vi "VI FID Konfig.vi"() -> ()   [LabVIEW 2020, in "ABB-EL3000.lvlib" / "FID.lvlib"]
uses:
  FID.lvlib
  CalGas Aufschaltung/Aufschaltung CalGas_ANZEIGE.ctl
  Visualisierungs Elemente/Auswahlfeld.ctl
  FID Kalibrierung/FID Kal Komponente.ctl
  Modus.ctl
  Visualisierungs Elemente/Zahlen-Ausgabefeld.ctl
  FID Kalibrierung/Aktionen FID Kal Komponente.ctl
  CalGas Aufschaltung/FGV CalGas Aktionen.ctl
  FT-IR/FGV FT-IR Gasliste Aktionen.ctl
  Aktion FGV Messwerte_F.ctl
  Messdaten/Aktionen FGV Messdaten.ctl
  Allgemeine VI/FGV Uras26 Aktion.ctl
  FID Kalibrierung/Aktion FID Allgemeindaten.ctl
  Aktion STY_MES.ctl
  Passwortverwaltung/FGV Passwort Aktion.ctl
  Analysator Definition/FGV Analysator Definition Aktionen.ctl
  FID Kalibrierung/FID Kalibrieren.ctl
  FT-IR/FGV FT-IR Parameter.vi
  Hangup Check/Hangup Main.vi
  Messdaten/Messdaten.lvlib
  CalGas Aufschaltung/CalGas Aufschaltung.lvlib
  FT-IR/FT-IR.lvlib
  Allgemein/allgemeine Sub-VIs.lvlib
  Analysator Definition/Analysator Definition.lvlib
  Passwortverwaltung/Passwort.lvlib
  FID Kalibrierung/FID Kalibrierung.lvlib
  Allgemeine VI/Allgemeine VI.lvlib
  Grafik/Grafik.lvlib
  Hangup Check/Hangup Check.lvlib
panel:
  out "Wert CH4 2":sgl caption="Kal. Wert THC:" format="%.1f"
  in  "Hang-Up Check":bool caption="Endpunkt"
  out "Roh Wert THC:":T1 format="%.1f"
  out "Response":string
  in  "Switching time":sgl caption="sec" min=0 format="%#.0f"
  in  "Mode":T2
  out "THC":string
  out "Mwert CH4":sgl format="%.1f"
  out "PMwert CH4":sgl format="%.1f"
  out "Wert CH4":sgl caption="Konzentration" format="%.1f"
  out "Graph CH4":waveform(dbl)[](graph)
  out "CH4":string
  out "Mwert 1THC":sgl format="%.1f"
  out "PMwert 1THC":sgl format="%.1f"
  out "Wert1 THC":sgl caption="Konzentration" format="%.1f"
  out "Graph1THC":waveform(dbl)[](graph)
  out "NMHC":string
  out "Mwert NMHC":sgl format="%.1f"
  out "PMwert NMHC":sgl format="%.1f"
  out "Wert NMHC":sgl caption="Konzentration" format="%.1f"
  out "MNHC":waveform(dbl)[](graph)
  in  "Endpunkt THC":bool
  in  "0-Punkt THC":bool
  in  "Kalidaten":bool
  in  "Endpunkt":bool
  in  "0-Punkt":bool
  in  "HC Messbereich":u16(ring)
  out "Wartungsbedarf":bool
  out "Funktionskontrolle":bool
  out "Ausfall":bool
  out "Flow Stellg":sgl caption="%" format="%#.1g"
  out "Durchfluss:":sgl format="%#.1f"
  out "Druck MGA":sgl caption="%" format="%#.1f"
  out "Druck MGE:":sgl caption="%" format="%#.1f"
  out "Brenngas:":sgl caption="%" format="%#.1f"
  out "Brennluft:":sgl caption="%" format="%#.1f"
  out "Messgaseingang":sgl caption="%" format="%#.1f"
  out "Detektor":sgl caption="%" format="%#.1f"
  out "Druck Messgasausgang:":sgl format="%#.1f"
  out "Druck Messgaseingang:":sgl format="%#.1f"
  out "Druck Brenngas H2/He:":sgl format="%#.1f"
  out "Druck Brennluft:":sgl format="%#.1f"
  out "Temperatur Flamme:":sgl format="%#.1f"
  out "Temperatur Messgaseingang:":sgl format="%#.1f"
  out "Temperatur Detektor:":sgl format="%.1f"
  in  "FID kalibrieren mit:":T3
  in  "Aufschaltung CalGas":T4 {"Aufschaltpunkt" items=["Filterblock", "Analysator direkt", "PNS", "Entnahme", "Gasdivider"]; "Kalibriergas" items=["Stickstoff"]}
  # "Konfiguration FID"
  # "Grafik"
  # "Hilfsgrößen"
  # "Temperaturen"
  # "Stellgröße"
  # "°C"
  # "°C"
  # "°C"
  # "hPa"
  # "hPa"
  # "hPa"
  # "hPa"
  # "l/h"
  # "Aufschaltung Kalibriergas"
  # "Kalibriergas"
  # "Aufschaltpunkt"
  # "Analysator"
  # "Modus (cutter)"
  # "±"
  # "x"
  # "±"
  # "x"
  # "±"
  # "x"
  # "Durchfluss"
  # "Druck"
  # "STATUS"
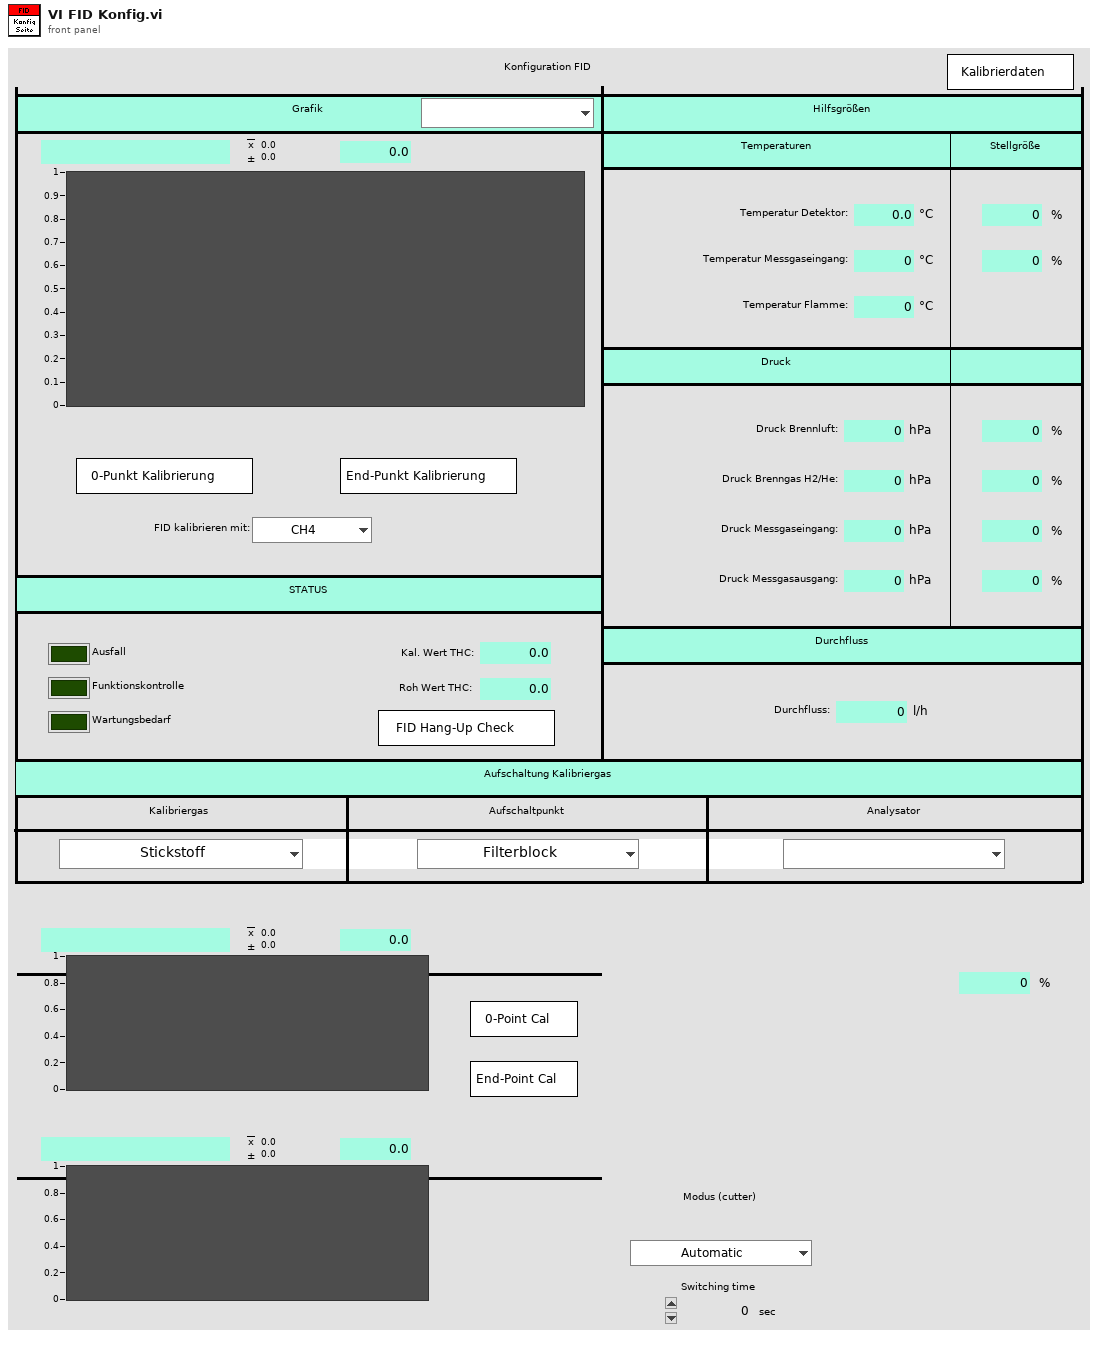
[diagram p1: front panel]
types:
  T1 = typedef "Zahlen-Ausgabefeld.ctl" = sgl
  T2 = typedef "ABB-EL3000.lvlib/FID.lvlib/Modus.ctl" = enum16{"Automatic", "CH4", "THC", "Efficienty measure", "Switching time"}
  T3 = typedef "ABB-EL3000.lvlib/FID.lvlib/FID Kalibrierung.lvlib/FID Kal Komponente.ctl" = enum16{"CH4", "C3H8"}
  T4 = typedef "CalGas Aufschaltung.lvlib/Aufschaltung CalGas_ANZEIGE.ctl" = cluster{"Kalibriergas":T5, "Aufschaltpunkt":T5, "Analysator":T5}
  T5 = typedef "Auswahlfeld.ctl" = u16
  T6 = typedef "ABB-EL3000.lvlib/FID.lvlib/FID Kalibrierung.lvlib/Aktionen FID Kal Komponente.ctl" = enum16{"lesen", "setzen", "laden", "speichern", "LIN"}
  T7 = typedef "ABB-EL3000.lvlib/FID.lvlib/FID Kalibrierung.lvlib/Aktion FID Allgemeindaten.ctl" = enum16{"lesen", "Mod", "Time", "laden", "speichern"}
  T8 = typedef "FT-IR.lvlib/FGV FT-IR Gasliste Aktionen.ctl" = enum16{"lesen", "Gasliste FT-IR", "Gasliste ausgelesen", "laden", "speichern", "löschen"}
  T9 = typedef "CalGas Aufschaltung.lvlib/FGV CalGas Aktionen.ctl" = enum16{"lesen", "Analysator Auswahl", "Def.CalGas", "Aufschaltung CalGas", "laden", "speichern", "KAL extrahieren"}
  T10 = typedef "String - Ausgabefeld.ctl" = string
  T11 = typedef "CalGas Aufschaltung.lvlib/Aufschaltung CalGas.ctl" = cluster{"Kalibriergas":T5, "Aufschaltpunkt":T12, "Analysator":T13}
  T12 = typedef "CalGas Aufschaltung.lvlib/Auswahl Aufschaltpunkt.ctl" = enum16{"über Filterblock", "Analysator direkt", "über PNS", "Entnahme", "Gasdivider"}
  T13 = typedef "CalGas Aufschaltung.lvlib/Auswahl Analysator.ctl" = enum16{"FT-IR", "FID", "PMA", "PMA/FID/FT-IR"}
  T14 = typedef "CalGas Aufschaltung.lvlib/Definition CalGas Anzeige.ctl" = cluster{"Namen":T15, "Werte":T17, "Werte 2":T17, "Einheit":T19, "Messbereiche":T20}
  T15 = typedef "CalGas Aufschaltung.lvlib/CalGas-Namen.ctl" = cluster{"Name":T16, "Name 2":T16, "Name 3":T16, "Name 4":T16, "Name 5":T16, "Name 6":T16, "Name 7":T16, "Name 8":T16, "Name 9":T16, "Name 10":T16, "Name 11":T16, "Name 12":T16}
  T16 = typedef "String - Eingabefeld.ctl" = string
  T17 = typedef "CalGas Aufschaltung.lvlib/CalGas-Werte.ctl" = cluster{"Konzentration 1":T18, "Konzentration 2":T18, "Konzentration 3":T18, "Konzentration 4":T18, "Konzentration 5":T18, "Konzentration 6":T18, "Konzentration 7":T18, "Konzentration 8":T18, "Konzentration 9":T18, "Konzentration 10":T18, "Konzentration 11":T18, "Konzentration 12":T18}
  T18 = typedef "Zahlen-Eingabefeld.ctl" = sgl
  T19 = typedef "CalGas Aufschaltung.lvlib/CalGas-Einheit.ctl" = cluster{"Einheit 1":T5, "Einheit 2":T5, "Einheit 3":T5, "Einheit 4":T5, "Einheit 5":T5, "Einheit 6":T5, "Einheit 7":T5, "Einheit 8":T5, "Einheit 9":T5, "Einheit 10":T5, "Einheit 11":T5, "Einheit 12":T5}
  T20 = typedef "CalGas Aufschaltung.lvlib/CalGas-Messbereiche.ctl" = cluster{"Messbereich 1":T5, "Messbereich 2":T5, "Messbereich 3":T5, "Messbereich 4":T5, "Messbereich 5":T5, "Messbereich 6":T5, "Messbereich 7":T5, "Messbereich 8":T5, "Messbereich 9":T5, "Messbereich 10":T5, "Messbereich 11":T5, "Messbereich 12":T5}
  T21 = typedef "Messdaten.lvlib/Aktionen FGV Messdaten.ctl" = enum16{"lesen", "schreiben", "löschen", "Mittelwerte", "Komponente"}
  T22 = typedef "ABB-EL3000.lvlib/Allgemeine VI.lvlib/FGV Uras26 Aktion.ctl" = enum16{"lesen", "CAL-Daten laden", "Messen", "Kalibrieren vorbereiten", "Kalibrieren", "CAL-Daten speichern", "Toleranz schreiben", "CAL-Daten kopieren"}
  T23 = typedef "ABB-EL3000.lvlib/FID.lvlib/Aktion FGV Messwerte_F.ctl" = enum16{"lesen", "Messwerte", "Messbereich", "Status", "Diagnose Werte"}
  T24 = typedef "Aktion STY_MES.ctl" = enum16{"lesen", "setze STY", "setze MES", "MODBUS schreiben"}
  T25 = typedef "Passwort.lvlib/FGV Passwort Aktion.ctl" = enum16{"prüfen", "setzen", "Initialisieren", "PW speichern", "lesen", "PW Änderung"}
  T26 = typedef "Analysator Definition.lvlib/FGV Analysator Definition Aktionen.ctl" = enum16{"lesen", "MB setzen", "MB KAL setzen", "laden"}
  T27 = typedef "ABB-EL3000.lvlib/FID.lvlib/FID Kalibrierung.lvlib/FID Kalibrieren.ctl" = enum16{"CH4 Nullpunkt", "THC Nullpunkt", "NMHC Nullpunkt", "CH4 Endpunkt", "THC Endpunkt", "NMHC Endpunkt"}
  T28 = cluster{"Temperatur Detektor":sgl, "STG Detektor":sgl, "Temperatur MGE":sgl, "STG MGE":sgl, "Druck Brennluft":sgl, "STG Brennluft":sgl, "Druck Brenngas":sgl, "STG Brenngas":sgl, "Druck MGE":sgl, "STG Druck MGE":sgl, "Druck MGA":sgl, "STG Druck MGA":sgl, "Flow":sgl, "Temperatur Flamme":sgl, "Temperatur NMHC":sgl, "STG NMHC":sgl}
  T29 = cluster{"Ausfall":bool, "Funktionskontrolle":bool, "Wartungsbedarf":bool}
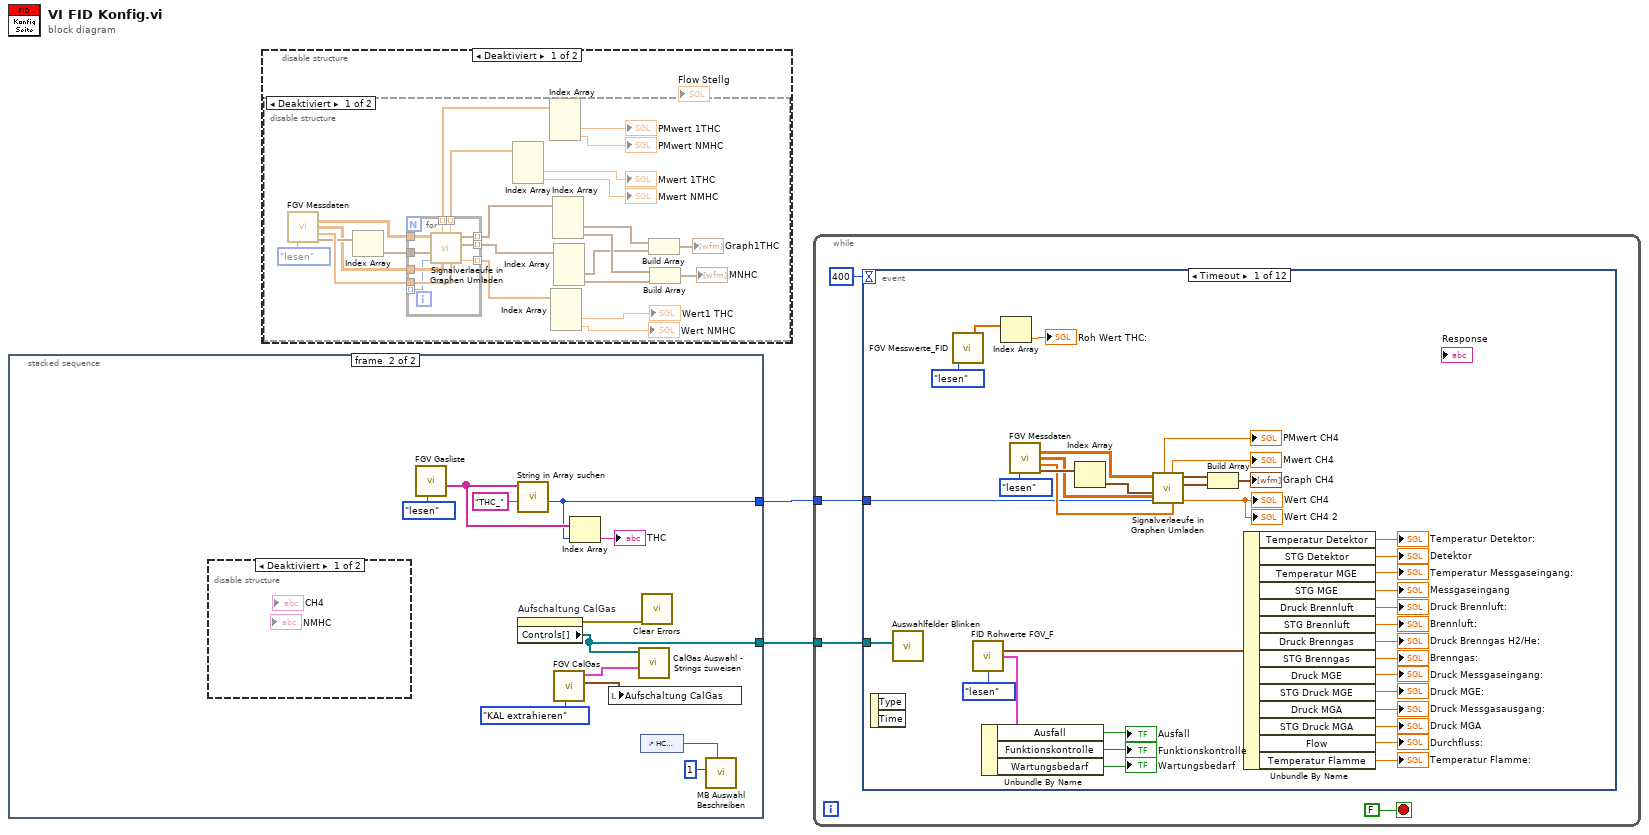
[diagram p0: block diagram]
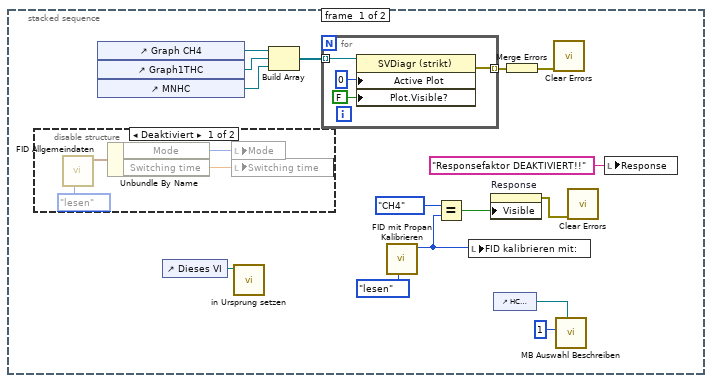
[diagram p2: hidden frame]
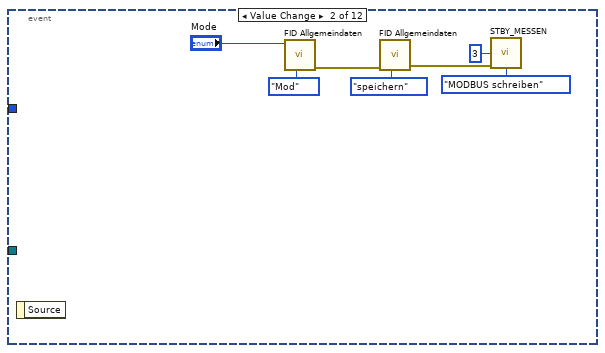
[diagram p7: hidden frame]
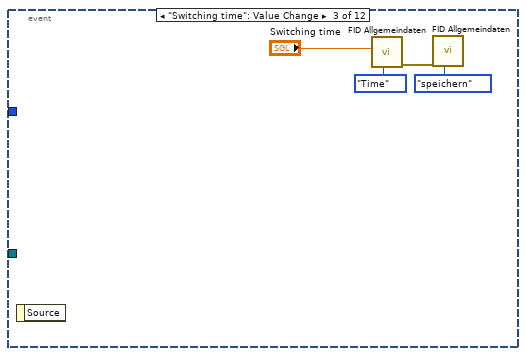
[diagram p8: hidden frame]
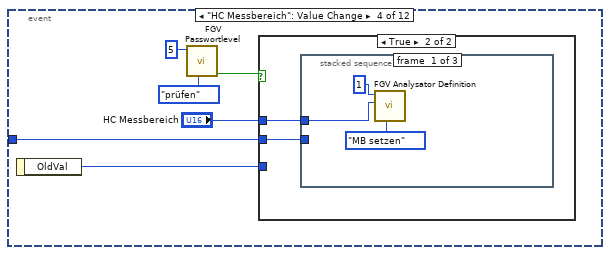
[diagram p9: hidden frame]
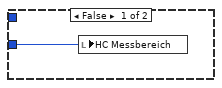
[diagram p10: hidden frame]
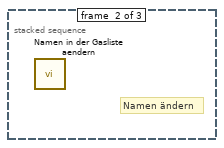
[diagram p11: hidden frame]
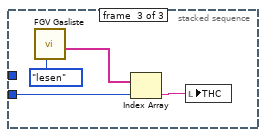
[diagram p12: hidden frame]
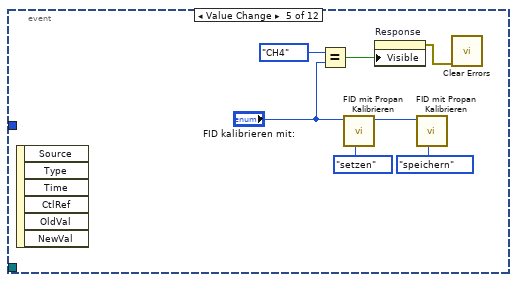
[diagram p13: hidden frame]
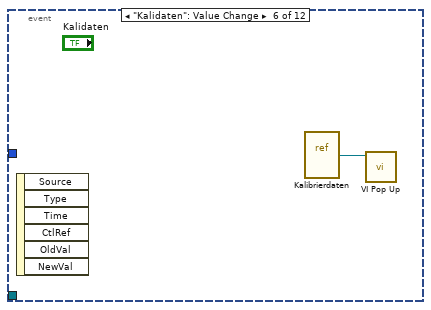
[diagram p14: hidden frame]
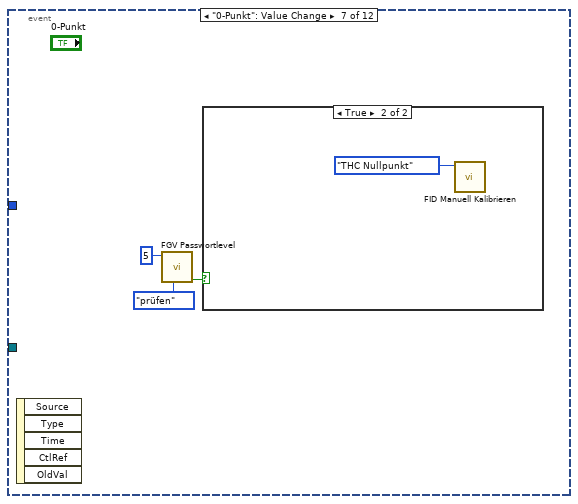
[diagram p15: hidden frame]
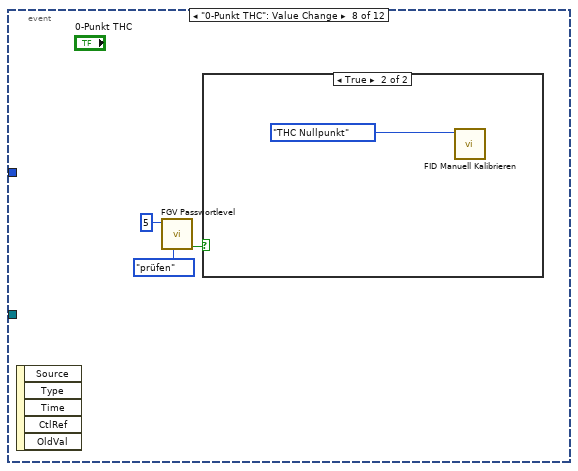
[diagram p17: hidden frame]
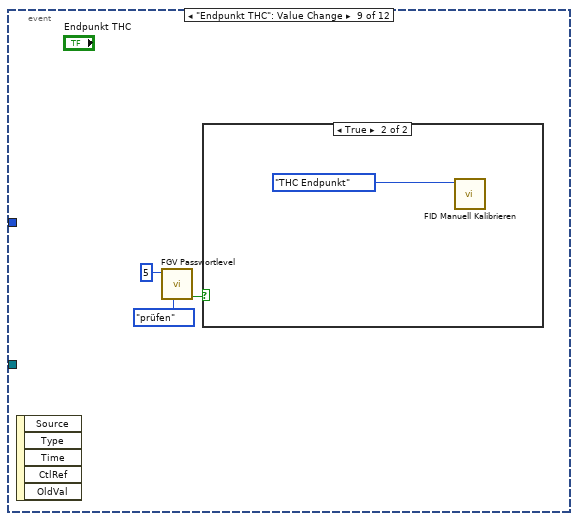
[diagram p19: hidden frame]
diagram:
  n1 = stacked-sequence {
    tunnel: [_ w34] -> w2
    tunnel: [_ w26] -> w1
    frame #0 {
      n2 = disable-structure shown="Deaktiviert" {
        frame Disabled {
          n3 = call "FID Allgemeindaten.vi"("Aktion"=Aktion_FID_Allgemeindaten."lesen") -> ("FID Allgemein"=w21:cluster{"Mode":T2, "Switching time":sgl})  [unwired: 9 in, 1 out]
          n4 = Unbundle By Name(w21) -> ("Mode"=w19:T2, "Switching time"=w18:sgl)
          n5 = local write "Mode"(w19) -> ()
          n6 = local write "Switching time"(w18) -> ()
        }
        frame Enabled {
        }
      }
      n7 = control-ref of="Graph CH4"() -> (w16:refnum<vi>)
      n8 = control-ref of="Graph1THC"() -> (w15:refnum<vi>)
      n9 = control-ref of="MNHC"() -> (w14:refnum<vi>)
      n10 = control-ref of="Dieses VI"() -> (w10:refnum<vi>)
      n11 = call "in Ursprung setzen.vi"("VI Referenz"=w10) -> ()  [unwired: 10 in, 1 out]
      n12 = Build Array(w16, w15, w14) -> (w13:refnum<vi>[])
      n13 = for {
        tunnel: w13 -> [w23] mode=indexing
        tunnel: [w22] -> w12 mode=indexing
        n14 = property class="SVDiagr (strikt)"(reference=w23, "Active Plot"=u32 0 ("Aktiver Plot"), "Plot.Visible?"=FALSE ("Plot.Sichtbar")) -> (error out=w22:errorcluster)  [unwired: 1 in, 1 out]
      }
      n15 = call "FID mit Propan Kalibrieren.vi"("Aktionen"=Aktionen_FID_Kal_Komponente."lesen") -> ("FID Kal Komponente"=w6:T3)  [unwired: 9 in, 1 out]
      n16 = Equal?(x=FID_Kal_Komponente."CH4", y=w6) -> (x = y?=w4:bool)
      n17 = local write "FID kalibrieren mit:"(w6) -> ()
      n18 = property on="Response" class="Str"("Visible"=w4) -> (error out=w3:errorcluster)  [unwired: 2 in, 1 out]
      n19 = control-ref of="HC Messbereich"() -> (w9:refnum<vi>)
      n20 = Merge Errors(w12) -> (w11:errorcluster)
      n21 = call <vilib>:"Clear Errors.vi"("error in (no error)"=w11) -> ()  [unwired: 5 in, 2 out]
      n22 = call "MB Auswahl Beschreiben.vi"("Auswahl Referenz"=w9, "Komponente"=1) -> ()  [unwired: 10 in]
      n23 = call <vilib>:"Clear Errors.vi"("error in (no error)"=w3) -> ()  [unwired: 5 in, 2 out]
      n24 = local write "Response"("Responsefaktor DEAKTIVIERT!!" ("Response")) -> ()
    }
    frame #1 {
      n25 = disable-structure shown="Deaktiviert" {
        frame Disabled {
        }
        frame Enabled {
        }
      }
      n26 = call "FGV Gasliste.vi"("Aktionen"=FGV_FT-IR_Gasliste_Aktionen."lesen") -> ("Aktuelle Gasliste gesamt"=w28:T10[])  [unwired: 8 in, 2 out]
      n27 = call "String in Array suchen.vi"("Nach String/Zeichen suchen (-)"="THC_", "String-Array"=w28) -> ("Index"=w26:i32)  [unwired: 7 in, 2 out]
      n28 = property on="Aufschaltung CalGas" class="Cluster (strikt)"() -> (error out=w33:errorcluster, "Controls[]"=w34:refnum<vi>[])  [unwired: 2 in, 1 out]
      n29 = call "FGV CalGas.vi"("Aktionen"=FGV_CalGas_Aktionen."KAL extrahieren") -> ("Aufschaltung CalGas"=w35:T11, "Def.CalGas"=w36:T14)  [unwired: 6 in, 3 out]
      n30 = Index Array(array=w28, index=w26) -> (element=→"THC":T10)
      n31 = local write "Aufschaltung CalGas"(w35) -> ()
      n32 = call "CalGas Auswahl - Strings zuweisen.vi"("Def.CalGas"=w36, "Aufschaltung CalGas"=w34) -> ()  [unwired: 9 in, 1 out]
      n33 = control-ref of="HC Messbereich"() -> (w32:refnum<vi>)
      n34 = call <vilib>:"Clear Errors.vi"("error in (no error)"=w33) -> ()  [unwired: 5 in, 2 out]
      n35 = call "MB Auswahl Beschreiben.vi"("Auswahl Referenz"=w32, "Komponente"=1) -> ()  [unwired: 10 in]
    }
  }
  n36 = disable-structure shown="Deaktiviert" {
    frame Disabled {
      n37 = disable-structure shown="Deaktiviert" {
        frame Disabled {
          n38 = call "FGV Messdaten.vi"("Aktionen"=Aktionen_FGV_Messdaten."lesen") -> ("Messdaten"=w62:sgl[][], "Mittelwertdaten"=w61:sgl[][], "Deviation"=w66:sgl[], "Zeitstempeln"=w64:timestamp[])  [unwired: 6 in, 5 out]
          n39 = Index Array(array=w64) -> (element=w65:timestamp)  [unwired: 1 in]
          n40 = for {
            tunnel: w66 -> [w76]
            tunnel: w65 -> [w75]
            tunnel: w62 -> [w74]
            tunnel: w61 -> [w73]
            tunnel: [w72] -> w59 mode=indexing
            tunnel: [w71] -> w57 mode=indexing
            tunnel: [w70] -> w51 mode=indexing
            tunnel: [w69] -> w54 mode=indexing
            tunnel: [w68] -> w55 mode=indexing
            tunnel: [w67] -> w60 mode=indexing
            n41 = call "Signalverlaeufe in Graphen Umladen.vi"("Deviation"=w76, "Mittelwertdaten"=w73, "Gas-Auswahl"=w67, "t0"=w75, "Werte"=w74) -> ("Konzentration"=w70:sgl, "Mittelwert"=w69:waveform(dbl), "Waveform"=w68:waveform(dbl), "aktuelle Mittelwert"=w71:sgl, "Deviation"=w72:sgl)  [unwired: 2 in]
          }
          n42 = Index Array(array=w57) -> (element #1=w56:sgl, element #2=→"Mwert 1THC":sgl, element #3=→"Mwert NMHC":sgl)  [unwired: 3 in]
          n43 = Index Array(array=w59) -> (element #1=w58:sgl, element #2=→"PMwert 1THC":sgl, element #3=→"PMwert NMHC":sgl)  [unwired: 3 in]
          n44 = Index Array(array=w51) -> (element #1=w50:sgl, element #2=→"Wert1 THC":sgl, element #3=→"Wert NMHC":sgl)  [unwired: 3 in]
          n45 = Index Array(array=w55) -> (element #1=w53:waveform(dbl), element #2=w49:waveform(dbl), element #3=w48:waveform(dbl))  [unwired: 3 in]
          n46 = Index Array(array=w54) -> (element #1=w52:waveform(dbl), element #2=w47:waveform(dbl), element #3=w46:waveform(dbl))  [unwired: 3 in]
          n47 = Build Array(w49, w47) -> (→"Graph1THC":waveform(dbl)[])
          n48 = Build Array(w48, w46) -> (→"MNHC":waveform(dbl)[])
        }
        frame Enabled {
        }
      }
    }
    frame Enabled {
    }
  }
  n49 = while {
    tunnel: w2 -> [w78]
    tunnel: w1 -> [w77]
    stop <- FALSE stop-if-true
    n50 = event shown="[0] Timeout" {
      selector: _ -> [_ _ _ _ _ _ _ _ _ _ _ _]
      dyn-events: _ -> [_ _ _ _ _ _ _ _ _ _ _ _]
      timeout: 400 -> [_ _ _ _ _ _ _ _ _ _ _ _]
      tunnel: w78 -> [w117 _ _ _ _ _ _ _ _ _ _ _]
      tunnel: w77 -> [w91 _ _ w129 _ _ _ _ _ _ _ _]
      event Timeout {
        n51 = event-data() -> ()  [unwired: 1 in, 2 out]
        n52 = call "Auswahlfelder Blinken.vi"("Controls[]"=w117) -> ()  [unwired: 11 in]
        n53 = call "FGV Messwerte_FID.vi"("Aktion"=FGV_Uras26_Aktion."lesen") -> ("Rohwerte"=w84:sgl[])  [unwired: 19 in, 7 out]
        n54 = call "FID Rohwerte FGV_F.vi"("Aktion"=Aktion_FGV_Messwerte_F."lesen") -> ("Diagnose Werte"=w116:T28, "Status"=w102:T29)  [unwired: 11 in, 2 out]
        n55 = Unbundle By Name(w102) -> ("Ausfall"=→"Ausfall":bool, "Funktionskontrolle"=→"Funktionskontrolle":bool, "Wartungsbedarf"=→"Wartungsbedarf":bool)
        n56 = Index Array(array=w84) -> (element=→"Roh Wert THC:":sgl)  [unwired: 1 in]
        n57 = call "FGV Messdaten.vi"("Aktionen"=Aktionen_FGV_Messdaten."lesen") -> ("Messdaten"=w95:sgl[][], "Mittelwertdaten"=w93:sgl[][], "Deviation"=w92:sgl[], "Zeitstempeln"=w97:timestamp[])  [unwired: 6 in, 5 out]
        n58 = Index Array(array=w97) -> (element=w94:timestamp)  [unwired: 1 in]
        n59 = call "Signalverlaeufe in Graphen Umladen.vi"("Deviation"=w92, "Mittelwertdaten"=w93, "Gas-Auswahl"=w91, "t0"=w94, "Werte"=w95) -> ("Konzentration"=→"Wert CH4" →"Wert CH4 2":sgl, "Mittelwert"=w87:waveform(dbl), "Waveform"=w88:waveform(dbl), "aktuelle Mittelwert"=→"Mwert CH4":sgl, "Deviation"=→"PMwert CH4":sgl)  [unwired: 2 in]
        n60 = Build Array(w88, w87) -> (→"Graph CH4":waveform(dbl)[])
        n61 = Unbundle By Name(w116) -> ("Temperatur Detektor"=→"Temperatur Detektor:":sgl, "STG Detektor"=→"Detektor":sgl, "Temperatur MGE"=→"Temperatur Messgaseingang:":sgl, "STG MGE"=→"Messgaseingang":sgl, "Druck Brennluft"=→"Druck Brennluft:":sgl, "STG Brennluft"=→"Brennluft:":sgl, "Druck Brenngas"=→"Druck Brenngas H2/He:":sgl, "STG Brenngas"=→"Brenngas:":sgl, "Druck MGE"=→"Druck Messgaseingang:":sgl, "STG Druck MGE"=→"Druck MGE:":sgl, "Druck MGA"=→"Druck Messgasausgang:":sgl, "STG Druck MGA"=→"Druck MGA":sgl, "Flow"=→"Durchfluss:":sgl, "Temperatur Flamme"=→"Temperatur Flamme:":sgl)
      }
      event Value Change {
        n62 = event-data() -> ()  [unwired: 1 in, 1 out]
        n63 = call "FID Allgemeindaten.vi"("Aktion"=Aktion_FID_Allgemeindaten."Mod", "Mode"="Mode") -> ("error out"=w121:errorcluster)  [unwired: 8 in, 1 out]
        n64 = call "FID Allgemeindaten.vi"("Aktion"=Aktion_FID_Allgemeindaten."speichern", "error in (no error)"=w121) -> ("error out"=w118:errorcluster)  [unwired: 8 in, 1 out]
        n65 = call "STBY_MESSEN.vi"("Case Nr."=3, "error in (no error)"=w118, "Aktion"=Aktion_STY_MES."MODBUS schreiben") -> ()  [unwired: 9 in, 4 out]
      }
      event "Switching time": Value Change {
        n66 = event-data() -> ()  [unwired: 1 in, 1 out]
        n67 = call "FID Allgemeindaten.vi"("Aktion"=Aktion_FID_Allgemeindaten."Time", "Switching time"="Switching time") -> ("error out"=w125:errorcluster)  [unwired: 8 in, 1 out]
        n68 = call "FID Allgemeindaten.vi"("Aktion"=Aktion_FID_Allgemeindaten."speichern", "error in (no error)"=w125) -> ()  [unwired: 8 in, 2 out]
      }
      event "HC Messbereich": Value Change {
        n69 = event-data() -> ("OldVal"=w134:u16)  [unwired: 1 in]
        n70 = call "FGV Passwortlevel.vi"("FGV Passwort Aktion"=FGV_Passwort_Aktion."prüfen", "geforderter Level"=i16 5) -> ("Freigabe"=w131:bool)  [unwired: 7 in, 2 out]
        n71 = case shown="True" w131 {
          tunnel: w134 -> [w135 _]
          tunnel: "HC Messbereich" -> [_ w137]
          tunnel: w129 -> [_ w136]
          frame False {
            n72 = local write "HC Messbereich"(w135) -> ()
          }
          frame True {
            n73 = stacked-sequence {
              tunnel: w137 -> [w138 _ _]
              tunnel: w136 -> [_ _ w141]
              frame #0 {
                n74 = call "FGV Analysator Definition.vi"("Aktionen"=FGV_Analysator_Definition_Aktionen."MB setzen", "Messbereich"=w138, "Komponente"=1) -> ()  [unwired: 4 in, 5 out]
              }
              frame #1 {
                # "Namen ändern"
                n75 = call "Namen in der Gasliste aendern.vi"() -> ()  [unwired: 12 in]
              }
              frame #2 {
                n76 = call "FGV Gasliste.vi"("Aktionen"=FGV_FT-IR_Gasliste_Aktionen."lesen") -> ("Aktuelle Gasliste gesamt"=w144:T10[])  [unwired: 8 in, 2 out]
                n77 = Index Array(array=w144, index=w141) -> (element=w142:T10)
                n78 = local write "THC"(w142) -> ()
              }
            }
          }
        }
      }
      event Value Change {
        n79 = event-data() -> ()  [unwired: 1 in, 6 out]
        n80 = Equal?(x=FID_Kal_Komponente."CH4", y="FID kalibrieren mit:") -> (x = y?=w147:bool)
        n81 = call "FID mit Propan Kalibrieren.vi"("Aktionen"=Aktionen_FID_Kal_Komponente."setzen", "FID Kal Komponente"="FID kalibrieren mit:") -> ("FID Kal Komponente"=w149:T3)  [unwired: 8 in, 1 out]
        n82 = property on="Response" class="Str"("Visible"=w147) -> (error out=w148:errorcluster)  [unwired: 2 in, 1 out]
        n83 = call "FID mit Propan Kalibrieren.vi"("Aktionen"=Aktionen_FID_Kal_Komponente."speichern", "FID Kal Komponente"=w149) -> ()  [unwired: 8 in, 2 out]
        n84 = call <vilib>:"Clear Errors.vi"("error in (no error)"=w148) -> ()  [unwired: 5 in, 2 out]
      }
      event "Kalidaten": Value Change {
        n85 = event-data() -> ()  [unwired: 1 in, 6 out]
        n86 = vi-ref "Kalibrierdaten.vi"() -> (w152:refnum<vi>)
        n87 = call "VI Pop Up.vi"("VI Referenz"=w152) -> ()  [unwired: 10 in, 1 out]
      }
      event "0-Punkt": Value Change {
        n88 = event-data() -> ()  [unwired: 1 in, 5 out]
        n89 = call "FGV Passwortlevel.vi"("FGV Passwort Aktion"=FGV_Passwort_Aktion."prüfen", "geforderter Level"=i16 5) -> ("Freigabe"=w153:bool)  [unwired: 7 in, 2 out]
        n90 = case shown="True" w153 {
          frame False {
          }
          frame True {
            n91 = call "FID Manuell Kalibrieren.vi"("Kalibrieren"=FID_Kalibrieren."THC Nullpunkt") -> ()  [unwired: 9 in, 2 out]
          }
        }
      }
      event "0-Punkt THC": Value Change {
        n92 = event-data() -> ()  [unwired: 1 in, 5 out]
        n93 = call "FGV Passwortlevel.vi"("FGV Passwort Aktion"=FGV_Passwort_Aktion."prüfen", "geforderter Level"=i16 5) -> ("Freigabe"=w157:bool)  [unwired: 7 in, 2 out]
        n94 = case shown="True" w157 {
          frame False {
          }
          frame True {
            n95 = call "FID Manuell Kalibrieren.vi"("Kalibrieren"=FID_Kalibrieren."THC Nullpunkt") -> ()  [unwired: 9 in, 2 out]
          }
        }
      }
      event "Endpunkt THC": Value Change {
        n96 = event-data() -> ()  [unwired: 1 in, 5 out]
        n97 = call "FGV Passwortlevel.vi"("FGV Passwort Aktion"=FGV_Passwort_Aktion."prüfen", "geforderter Level"=i16 5) -> ("Freigabe"=w161:bool)  [unwired: 7 in, 2 out]
        n98 = case shown="True" w161 {
          frame False {
          }
          frame True {
            n99 = call "FID Manuell Kalibrieren.vi"("Kalibrieren"=FID_Kalibrieren."THC Endpunkt") -> ()  [unwired: 9 in, 2 out]
          }
        }
      }
      event "Endpunkt": Value Change {
        n100 = event-data() -> ()  [unwired: 1 in, 1 out]
        n101 = call "FGV Passwortlevel.vi"("FGV Passwort Aktion"=FGV_Passwort_Aktion."prüfen", "geforderter Level"=i16 5) -> ("Freigabe"=w165:bool)  [unwired: 7 in, 2 out]
        n102 = case shown="True" w165 {
          frame False {
          }
          frame True {
            n103 = call "FID Manuell Kalibrieren.vi"("Kalibrieren"=FID_Kalibrieren."THC Endpunkt") -> ()  [unwired: 9 in, 2 out]
          }
        }
      }
      event Value Change {
        n104 = event-data() -> ()  [unwired: 1 in, 2 out]
        n105 = call "FGV CalGas.vi"("Aktionen"=FGV_CalGas_Aktionen."Aufschaltung CalGas", "Aufschaltung CalGas"="Aufschaltung CalGas") -> ()  [unwired: 5 in, 5 out]
      }
      event "Hang-Up Check": Value Change {
        n106 = event-data() -> ()  [unwired: 1 in, 6 out]
        n107 = vi-ref "Hangup Check.lvlib:Hangup Main.vi"() -> (w171:refnum<vi>)
        n108 = call "VI Pop Up.vi"("VI Referenz"=w171) -> ()  [unwired: 10 in, 1 out]
      }
    }
  }
